vi "SetMultiLineColor(Refresh).vi"(7 "色指定":cluster{"背景色":u32, "文字色":u32}, 8 "Error In":errorcluster caption="エラー入力", 9 "長さ(1)":i32=1, 10 "開始行(0)":i32, 11 "Tbl refnum":refnum<vi>) -> (0 "Error Out":errorcluster caption="エラー出力", 3 "Tbl refnum出力":refnum<vi>)   [LabVIEW 2014]
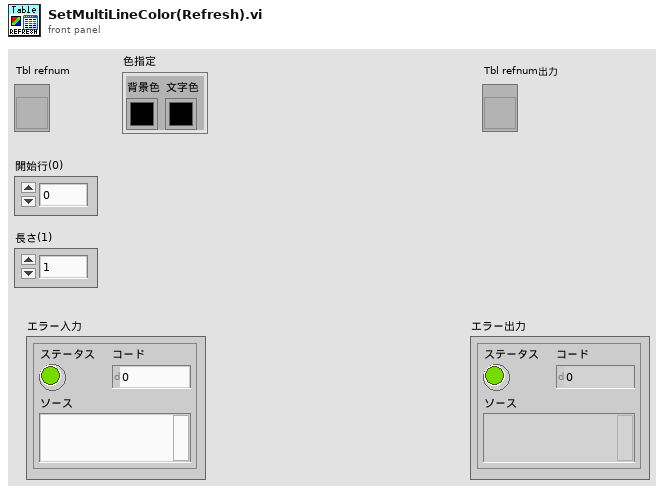
[diagram p1: front panel]
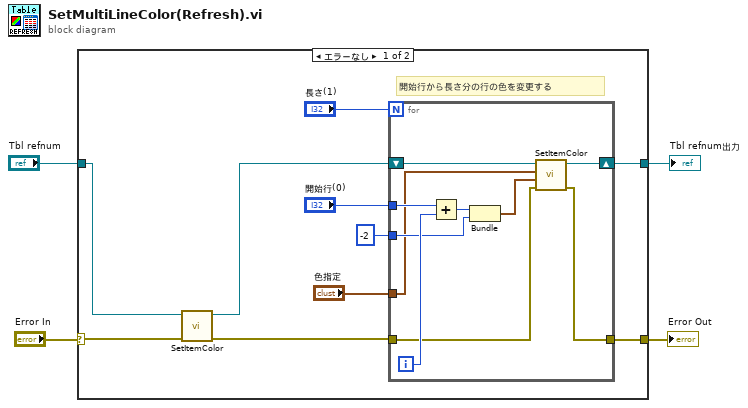
[diagram p0: block diagram]
diagram:
  n1 = case shown="エラーなし" "Error In" {
    selector: "Error In" -> [w8 w26]
    tunnel: [w10 w26] -> w3
    tunnel: "Tbl refnum" -> [w6 w25]
    tunnel: [w9 w25] -> w1
    frame No Error {
      # "開始行から長さ分の行の色を変更する"
      n2 = call "SetItemColor.vi"("エラー入力(エラーなし)"=w8, "Tbl refnum"=w6) -> ("エラー出力"=w7:errorcluster, "Tbl refnum出力"=w5:refnum<vi>)  [unwired: 8 in]
      n3 = for {
        N: "長さ(1)" -> [_]
        tunnel: "開始行(0)" -> [w24]
        tunnel: -2 -> [w21]
        tunnel: "色指定" -> [w19]
        tunnel: w7 -> [w18]
        tunnel: [w17] -> w10
        shift-right: [w15] -> w9
        shift-left: w5 -> [w16]
        i -> [w23]
        n4 = Add(x=w24, y=w23) -> (x+y=w22:i32)
        n5 = Bundle(w22, w21) -> (w20:cluster{i32, i32})  [unwired: 1 in]
        n6 = call "SetItemColor.vi"("エラー入力(エラーなし)"=w18, "行列指定"=w20, "色指定"=w19, "Tbl refnum"=w16) -> ("エラー出力"=w17:errorcluster, "Tbl refnum出力"=w15:refnum<vi>)  [unwired: 6 in]
      }
    }
    frame Error {
    }
  }
  "Error Out" <- w3
  "Tbl refnum出力" <- w1
